vi "Get Active Comparision Function.vi"(0 "Comparison Functions in":refnum<class "Comparison Functions.lvclass">, 11 "error in (no error)":errorcluster) -> (4 "Comparison Functions out":refnum<class "Comparison Functions.lvclass">, 6 "Function List":T1, 15 "error out":errorcluster)   [LabVIEW 2019, in "Comparison Functions.lvclass"]
uses:
  Comparison Functions.lvclass
  C:/Users/Patrick/Documents/GitHub/LabVIEW-Script-Language/source code/LSL components/functions/functionsbase/functionbase.lvclass
  Function List.ctl
  functionsbase/functionbase.lvclass
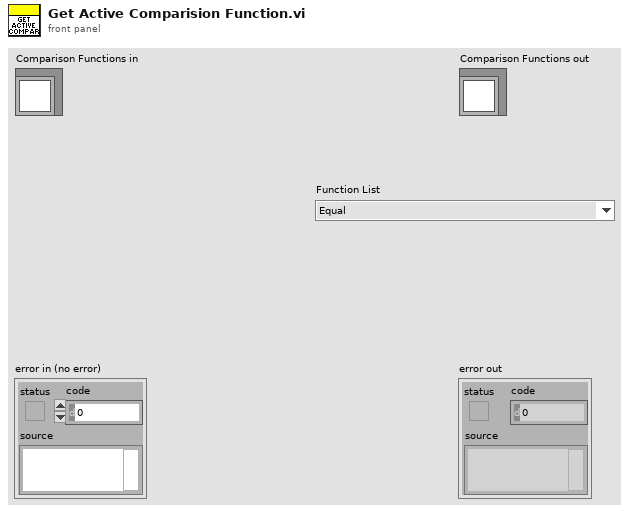
[diagram p1: front panel]
types:
  T1 = typedef "Comparison Functions.lvclass/Function List.ctl" = enum16{"Equal", "Not Equal", "Greater Than", "Less Than", "Greater Than Or Equal", "Lesser Than Or Equal", "Equal To Zero", "Select One", "In Range", "Empty Array", "Empty String", "Not A Number"}
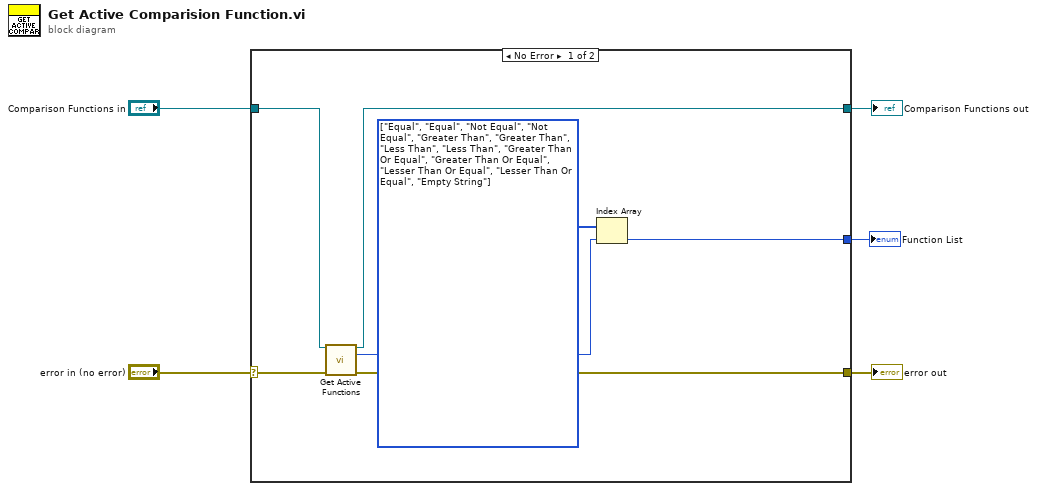
[diagram p0: block diagram]
diagram:
  n1 = case shown="No Error" "error in (no error)" {
    selector: "error in (no error)" -> [w12 w14]
    tunnel: [w11 w14] -> w4
    tunnel: [w9 w13] -> w2
    tunnel: "Comparison Functions in" -> [w10 w13]
    tunnel: [w6 _] -> w1
    frame No Error {
      w8 = T1[] [enum."Equal", enum."Equal", enum."Not Equal", enum."Not Equal", enum."Greater Than", enum."Greater Than", enum."Less Than", enum."Less Than", enum."Greater Than Or Equal", enum."Greater Than Or Equal", enum."Lesser Than Or Equal", enum."Lesser Than Or Equal", enum."Empty String"] items=["Equal", "Not Equal", "Greater Than", "Less Than", "Greater Than Or Equal", "Lesser Than Or Equal", "Equal To Zero", "Select One", "In Range", "Empty Array", "Empty String", "Not A Number"]
      n2 = call "Get Active Functions.vi"("functionbase in"=w10, "error in (no error)"=w12) -> ("functionbase out"=w9:refnum<class "Comparison Functions.lvclass">, "Syntax Index"=w7:i32, "error out"=w11:errorcluster)  [unwired: 11 in]
      n3 = Index Array(array=w8, index=w7) -> (element=w6:T1)
    }
    frame Error {
    }
  }
  "error out" <- w4
  "Comparison Functions out" <- w2
  "Function List" <- w1
